vi "FP_SubPanel_Size to Largest Decoration_.vi"(8 "Error":errorcluster, 9 "Border Spacing":i16=-2, 10 "Decoration Index":i32, 11 "VI Ref":refnum<vi>) -> (0 "Error Out":errorcluster, 1 "Bounds Out":T1, 2 "Position Out":T2, 3 "VI Ref Out":refnum<vi>)   [LabVIEW 2020]
uses:
  <vilib>/Utility/miscctls.llb/LVPositionTypeDef.ctl
  <vilib>/Utility/miscctls.llb/LVBoundsTypeDef.ctl
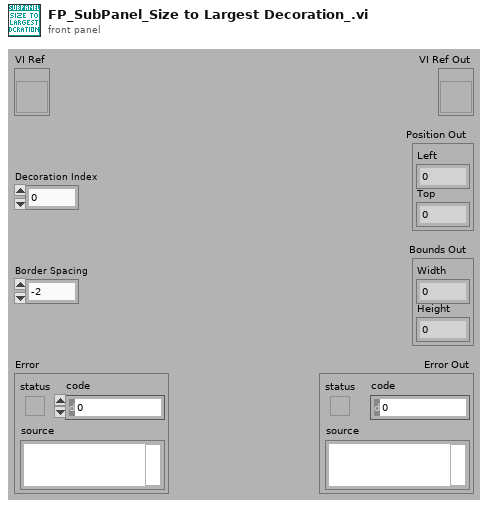
[diagram p1: front panel]
types:
  T1 = typedef "LVBoundsTypeDef.ctl" = cluster{"Width":u32, "Height":u32}
  T2 = typedef "LVPositionTypeDef.ctl" = cluster{"Left":i32, "Top":i32}
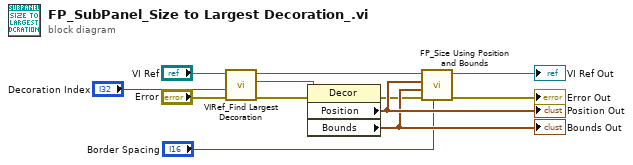
[diagram p0: block diagram]
diagram:
  n1 = call "VIRef_Find Largest Decoration.vi"("Error"="Error", "Decoration index"="Decoration Index", "VI's Ref"="VI Ref") -> ("Error Out"=w7:errorcluster, "Decor Refnum Out"=w11:refnum<vi>, "Calling VI's Ref Out"=w10:refnum<vi>)  [unwired: 2 in, 4 out]
  n2 = property class="Decor"(reference=w11, error in=w7) -> (error out=w6:errorcluster, "Position"=w9:T2, "Bounds"=w8:T1)  [unwired: 1 out]
  "Position Out" <- w9
  "Bounds Out" <- w8
  n3 = call "FP_Size Using Position and Bounds.vi"("Border Spacing"="Border Spacing", "Error"=w6, "Bounds"=w8, "Position"=w9, "VI"=w10) -> ("Error Out"=→"Error Out":errorcluster, "VI Out"=→"VI Ref Out":refnum<vi>)  [unwired: 4 in, 1 out]
